vi "Three_Tote_Dashboard_Values.vi"(11 "3_Tote_Enable":bool=TRUE) -> ()   [LabVIEW 2014]
uses:
  General_VI/Global Var.vi
  <vilib>/Rock Robotics/Network Tables/SD Read Number.vi
panel:
  in  "Time _To_Drive_1_Tote":i32=8000
  in  "Extend_Flipper_Time":i32=500
  in  "Open_Infeed_time":i32=800
  # "Static Tunning Values"
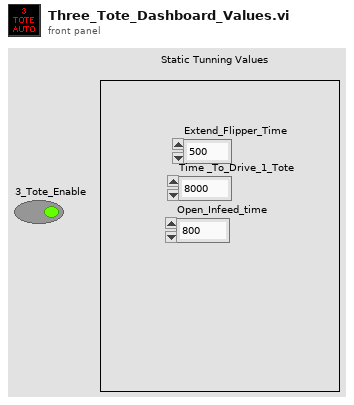
[diagram p1: front panel]
types:
  T1 = cluster{"Open_Infeed_time":i32, "Extend_Flipper_Time":i32, "Time _To_Drive_1_Tote":i32}
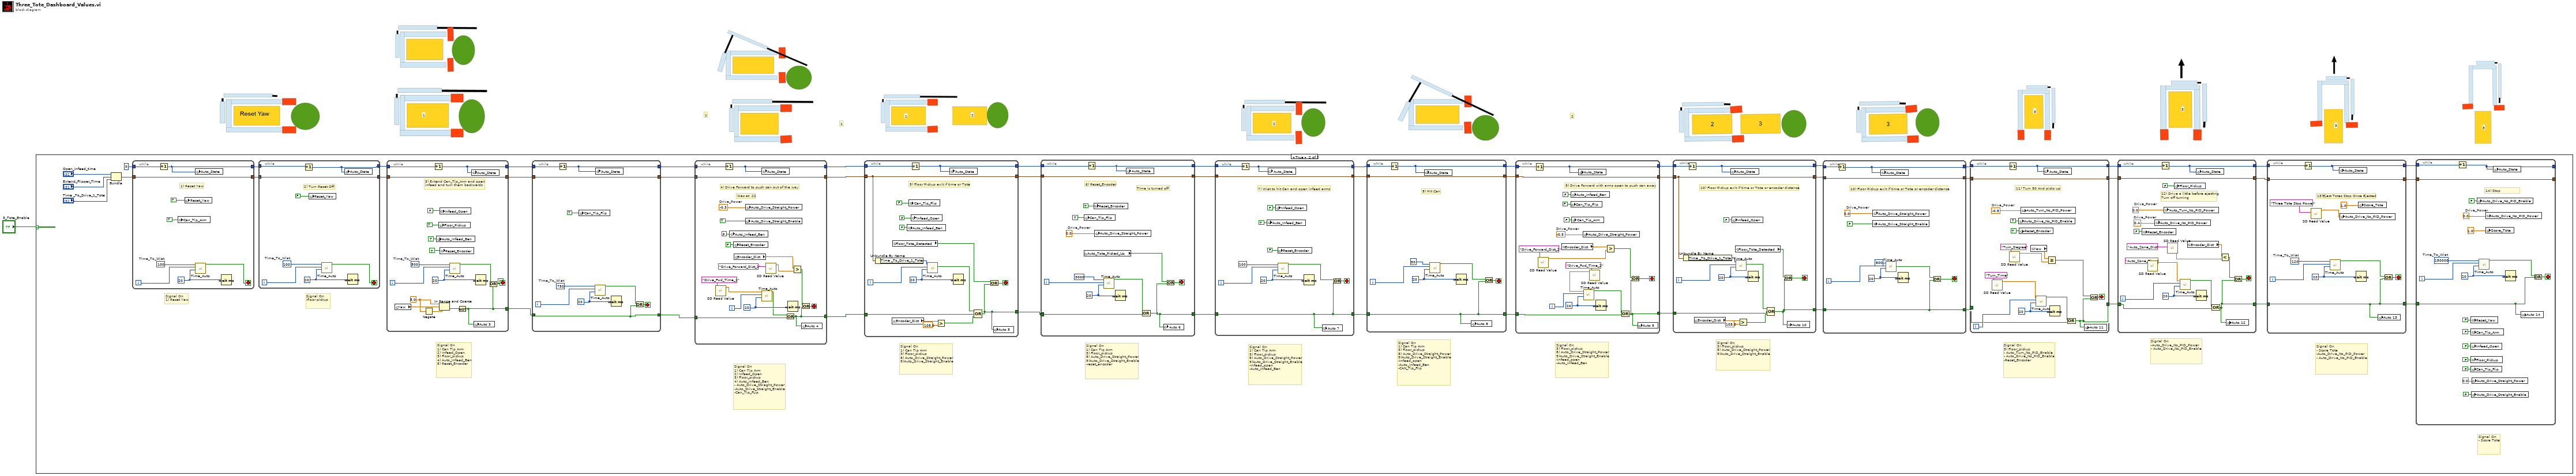
[diagram p0: block diagram]
diagram:
  # "3"
  # "3"
  # "3"
  # "3"
  # "2"
  # "2"
  # "2"
  # "1"
  # "1"
  # "1"
  # "1"
  n1 = case shown="True" "3_Tote_Enable" {
    frame False {
    }
    frame True {
      # "Signal On\n1) Can Tip Arm\n2) Infeed_Open\n3) Floor_pickup\n4) Auto_Infeed_Ben\n- Auto_Drive_Striaght_Power\n-Auto_Drive_Straight_Enable\n-Can_Tip_FLip"
      # "Signal On\n- Score Tote"
      # "Signal On\n- Score Tote\n-Auto_Drive_No_PID_Power\n- Auto_Drive_No_PID_Enable"
      # "Signal On\n-Auto_Drive_No_PID_Power\n- Auto_Drive_No_PID_Enable"
      # "Signal On\n3) Floor_pickup\n- Auto_Turn_No_PID_Enable\n- Auto_Drive_No_PID_Enable\n-Reset_Encoder"
      # "Signal On\n3) Floor_pickup\n8) Auto_Drive_Straight_Power\n9)Auto_Drive_Straight_Enable"
      # "Signal On\n3) Floor_pickup\n8) Auto_Drive_Straight_Power\n9)Auto_Drive_Straight_Enable\n-Infeed_open\n-Auto_Infeed_Ben"
      # "Signal On\n1) Can Tip Arm\n3) Floor_pickup\n8) Auto_Drive_Straight_Power\n9)Auto_Drive_Straight_Enable\n-Infeed_open\n-Auto_Infeed_Ben\n-CAN_Tip_Flip"
      # "Signal On\n1) Can Tip Arm\n3) Floor_pickup\n8) Auto_Drive_Straight_Power\n9)Auto_Drive_Straight_Enable\n-Infeed_open\n-Auto_Infeed_Ben"
      # "Signal On\n1) Can Tip Arm\n3) Floor_pickup\n8) Auto_Drive_Straight_Power\n9)Auto_Drive_Straight_Enable\n-reset_encoder"
      # "Signal On\n1) Can Tip Arm\n3) Floor_pickup\n8) Auto_Drive_Straight_Power\n9)Auto_Drive_Straight_Enable"
      # "Signal On\n1) Can Tip Arm\n2) Infeed_Open\n3) Floor_pickup\n4) Auto_Infeed_Ben\n5) Reset_Encoder"
      # "Signal On\n-floor pickup"
      # "Signal On\n1) Reset Yaw"
      n2 = Bundle("Open_Infeed_time"="Open_Infeed_time", "Extend_Flipper_Time"="Extend_Flipper_Time", "Time _To_Drive_1_Tote"="Time _To_Drive_1_Tote") -> (w39:T1)  [unwired: 1 in]
      n3 = while {
        tunnel: 0 -> [w271]
        tunnel: [w270] -> w48
        tunnel: w39 -> [w272]
        tunnel: [w272] -> w38
        i -> [w275]
        stop <- w277 stop-if-true
        w276 = u32 20 ("milliseconds to wait")
        w274 = 100  # Time_To_Wiat
        # "1) Reset Yaw"
        n4 = Increment(x=w271) -> (x+1=w270:i32)
        n5 = global write "Global Var.vi" "Can_Tip_Arm"(TRUE) -> ()
        n6 = global write "Global Var.vi" "Reset_Yaw"(TRUE) -> ()
        n7 = global write "Global Var.vi" "Auto_State"(w270) -> ()
        n8 = call "Time_Auto.vi"("Sample_Time"=w276, "Counter"=w275, "Time_to_wait"=w274) -> ("Boolean"=w277:bool)  [unwired: 8 in]
        n9 = Wait (ms)(milliseconds to wait=w276) -> ()  [unwired: 1 out]
      }
      n10 = while {
        tunnel: w48 -> [w262]
        tunnel: [w261] -> w47
        tunnel: w38 -> [w263]
        tunnel: [w263] -> w37
        i -> [w266]
        stop <- w268 stop-if-true
        w267 = u32 20 ("milliseconds to wait")
        w265 = 100  # Time_To_Wiat
        # "2) Turn Reset Off"
        n11 = Increment(x=w262) -> (x+1=w261:i32)
        n12 = global write "Global Var.vi" "Reset_Yaw"(FALSE) -> ()
        n13 = call "Time_Auto.vi"("Sample_Time"=w267, "Counter"=w266, "Time_to_wait"=w265) -> ("Boolean"=w268:bool)  [unwired: 8 in]
        n14 = global write "Global Var.vi" "Auto_State"(w261) -> ()
        n15 = Wait (ms)(milliseconds to wait=w267) -> ()  [unwired: 1 out]
      }
      n16 = while {
        tunnel: w47 -> [w256]
        tunnel: [w255] -> w11
        tunnel: w37 -> [w257]
        tunnel: [w257] -> w12
        tunnel: [w245] -> w14
        i -> [w259]
        stop <- w247 stop-if-true
        w251 = 5.0 ("upper limit")
        w260 = u32 20 ("milliseconds to wait")
        w258 = 500  # Time_To_Wiat
        # "3) Extend Can_Tip_Arm and open \ninfeed and turn them backwards"
        n17 = global read "Global Var.vi" "Yaw"() -> (w253:dbl)
        n18 = Negate(x=w251) -> (-x=w252:dbl)
        n19 = Increment(x=w256) -> (x+1=w255:i32)
        n20 = global write "Global Var.vi" "Auto_Infeed_Ben"(TRUE) -> ()
        n21 = global write "Global Var.vi" "Floor_Pickup"(TRUE) -> ()
        n22 = In Range and Coerce(upper limit=w251, x=w253, lower limit=w252) -> (In Range?=w250:bool)  [unwired: 1 out]
        n23 = global write "Global Var.vi" "Infeed_Open"(FALSE) -> ()
        n24 = global write "Global Var.vi" "Reset_Encoder"(TRUE) -> ()
        n25 = call "Time_Auto.vi"("Sample_Time"=w260, "Counter"=w259, "Time_to_wait"=w258) -> ("Boolean"=w246:bool)  [unwired: 8 in]
        n26 = Not(x=w250) -> (.not. x?=w245:bool)
        n27 = global write "Global Var.vi" "Auto_State"(w255) -> ()
        n28 = global write "Global Var.vi" "Auto 3"(w245) -> ()
        n29 = Wait (ms)(milliseconds to wait=w260) -> ()  [unwired: 1 out]
        n30 = Or(x=w246, y=w245) -> (x .or. y?=w247:bool)
      }
      n31 = while {
        tunnel: w11 -> [w66]
        tunnel: [w65] -> w10
        tunnel: w12 -> [w67]
        tunnel: [w67] -> w9
        tunnel: w14 -> [w61]
        tunnel: [w61] -> w13
        i -> [w69]
        stop <- w64 stop-if-true
        w70 = u32 20 ("milliseconds to wait")
        w68 = 750  # Time_To_Wiat
        n32 = Increment(x=w66) -> (x+1=w65:i32)
        n33 = global write "Global Var.vi" "Can_Tip_Flip"(TRUE) -> ()
        n34 = call "Time_Auto.vi"("Sample_Time"=w70, "Counter"=w69, "Time_to_wait"=w68) -> ("Boolean"=w62:bool)  [unwired: 8 in]
        n35 = global write "Global Var.vi" "Auto_State"(w65) -> ()
        n36 = Wait (ms)(milliseconds to wait=w70) -> ()  [unwired: 1 out]
        n37 = Or(x=w62, y=w61) -> (x .or. y?=w64:bool)
      }
      n38 = while {
        tunnel: w10 -> [w240]
        tunnel: [w239] -> w33
        tunnel: w9 -> [w241]
        tunnel: [w241] -> w32
        tunnel: w13 -> [w233]
        tunnel: [w230] -> w31
        i -> [w242]
        stop <- w232 stop-if-true
        w238 = -0.3  # Drive_Power
        w243 = u32 20 ("milliseconds to wait")
        # "Was at .22"
        # "4) Drive Forward to push can out of the way"
        n39 = call-poly <vilib>:"SD Read Value.vi"("Name"="Drive_Fwd_Time_1") -> ("Numeric"=w225:dbl)  [unwired: 8 in, 2 out]
        n40 = Increment(x=w240) -> (x+1=w239:i32)
        n41 = global write "Global Var.vi" "Auto_Infeed_Ben"(FALSE) -> ()
        n42 = global write "Global Var.vi" "Reset_Encoder"(FALSE ("Reset_Encoder")) -> ()
        n43 = global read "Global Var.vi" "Encoder_Dist"() -> (w235:dbl)
        n44 = global write "Global Var.vi" "Auto_Drive_Straight_Enable"(TRUE) -> ()
        n45 = global write "Global Var.vi" "Auto_Drive_Straight_Power"(w238) -> ()
        n46 = call "Time_Auto.vi"("Sample_Time"=w243, "Counter"=w242, "Time_to_wait"=w225) -> ("Boolean"=w234:bool)  [unwired: 8 in]
        n47 = global write "Global Var.vi" "Auto_State"(w239) -> ()
        n48 = call-poly <vilib>:"SD Read Value.vi"("Name"="Drive_Forward_Dist_1") -> ("Numeric"=w227:dbl)  [unwired: 8 in, 2 out]
        n49 = Or(x=w234, y=w233) -> (x .or. y?=w230:bool)
        n50 = Wait (ms)(milliseconds to wait=w243) -> ()  [unwired: 1 out]
        n51 = Greater?(x=w235, y=w227) -> (0:w231:bool)
        n52 = Or(x=w231, y=w230) -> (x .or. y?=w232:bool)
        n53 = global write "Global Var.vi" "Auto 4"(w230) -> ()
      }
      n54 = while {
        tunnel: w33 -> [w222]
        tunnel: [w221] -> w30
        tunnel: w32 -> [w220]
        tunnel: [w220] -> w29
        tunnel: w31 -> [w218]
        tunnel: [w208] -> w2
        i -> [w223]
        stop <- w214 stop-if-true
        w224 = u32 20 ("milliseconds to wait")
        # "5) Floor Pickup exit if time or Tote"
        n55 = Unbundle By Name(w220) -> ("Time _To_Drive_1_Tote"=w219:i32)
        n56 = global read "Global Var.vi" "Encoder_Dist"() -> (w212:dbl)
        n57 = global read "Global Var.vi" "Floor_Tote_Detected"() -> (w213:bool)
        n58 = global write "Global Var.vi" "Auto_Infeed_Ben"(FALSE) -> ()
        n59 = global write "Global Var.vi" "Can_Tip_Flip"(FALSE) -> ()
        n60 = Increment(x=w222) -> (x+1=w221:i32)
        n61 = global write "Global Var.vi" "Infeed_Open"(FALSE) -> ()
        n62 = call "Time_Auto.vi"("Sample_Time"=w224, "Counter"=w223, "Time_to_wait"=w219) -> ("Boolean"=w217:bool)  [unwired: 8 in]
        n63 = Greater?(x=w212, y=105.0) -> (0:w211:bool)
        n64 = global write "Global Var.vi" "Auto_State"(w221) -> ()
        n65 = Wait (ms)(milliseconds to wait=w224) -> ()  [unwired: 1 out]
        n66 = Compound Arithmetic op=OR(w217, w218, w211) -> (w208:bool)
        n67 = Or(x=w213, y=w208) -> (x .or. y?=w214:bool)
        n68 = global write "Global Var.vi" "Auto 5"(w208) -> ()
      }
      n69 = while {
        tunnel: w30 -> [w101]
        tunnel: [w100] -> w15
        tunnel: w29 -> [w99]
        tunnel: [w99] -> w22
        tunnel: w2 -> [_]
        tunnel: [w91] -> w28
        tunnel: w2 -> [w92]
        i -> [w102]
        stop <- w98 stop-if-true
        w94 = 0.0  # Drive_Power
        w103 = u32 20 ("milliseconds to wait")
        # "TIme is turned off"
        # "6) Reset_Encoder"
        n70 = global read "Global Var.vi" "Auto_Tote_Picked_Up"() -> (w95:bool)
        n71 = global write "Global Var.vi" "Can_Tip_Flip"(TRUE) -> ()
        n72 = Increment(x=w101) -> (x+1=w100:i32)
        n73 = global write "Global Var.vi" "Reset_Encoder"(TRUE) -> ()
        n74 = global write "Global Var.vi" "Auto_Drive_Straight_Power"(w94) -> ()
        n75 = call "Time_Auto.vi"("Sample_Time"=w103, "Counter"=w102, "Time_to_wait"=3000) -> ("Boolean"=w93:bool)  [unwired: 8 in]
        n76 = Wait (ms)(milliseconds to wait=w103) -> ()  [unwired: 1 out]
        n77 = global write "Global Var.vi" "Auto_State"(w100) -> ()
        n78 = Compound Arithmetic op=OR(w93, w92) -> (w91:bool)
        n79 = global write "Global Var.vi" "Auto 6"(w91) -> ()
        n80 = Or(x=w95, y=w91) -> (x .or. y?=w98:bool)
      }
      n81 = while {
        tunnel: [w205] -> w46
        tunnel: w28 -> [w196]
        tunnel: [w196] -> w27
        tunnel: w22 -> [w198]
        tunnel: [w198] -> w21
        tunnel: w15 -> [w197]
        i -> [w206]
        stop <- w203 stop-if-true
        w207 = u32 20 ("milliseconds to wait")
        # "7) Wiat to hit Can and open infeed arms"
        n82 = Increment(x=w197) -> (x+1=w205:i32)
        n83 = global write "Global Var.vi" "Auto_Infeed_Ben"(TRUE) -> ()
        n84 = global write "Global Var.vi" "Auto_State"(w205) -> ()
        n85 = global write "Global Var.vi" "Infeed_Open"(FALSE ("Infeed_Open")) -> ()
        n86 = global write "Global Var.vi" "Reset_Encoder"(FALSE) -> ()
        n87 = call "Time_Auto.vi"("Sample_Time"=w207, "Counter"=w206, "Time_to_wait"=100) -> ("Boolean"=w202:bool)  [unwired: 8 in]
        n88 = Wait (ms)(milliseconds to wait=w207) -> ()  [unwired: 1 out]
        n89 = global write "Global Var.vi" "Auto 7"(w196) -> ()
        n90 = Or(x=w202, y=w196) -> (x .or. y?=w203:bool)
      }
      n91 = while {
        tunnel: w46 -> [w193]
        tunnel: [w192] -> w26
        tunnel: w27 -> [w187]
        tunnel: [w187] -> w24
        tunnel: w21 -> [w189]
        tunnel: [w189] -> w20
        i -> [w194]
        stop <- w191 stop-if-true
        w195 = u32 20 ("milliseconds to wait")
        # "8) HIt Can"
        n92 = Increment(x=w193) -> (x+1=w192:i32)
        n93 = global write "Global Var.vi" "Auto_State"(w192) -> ()
        n94 = call "Time_Auto.vi"("Sample_Time"=w195, "Counter"=w194, "Time_to_wait"=50) -> ("Boolean"=w190:bool)  [unwired: 8 in]
        n95 = Wait (ms)(milliseconds to wait=w195) -> ()  [unwired: 1 out]
        n96 = global write "Global Var.vi" "Auto 8"(w187) -> ()
        n97 = Or(x=w190, y=w187) -> (x .or. y?=w191:bool)
      }
      n98 = while {
        tunnel: [w86] -> w25
        tunnel: w26 -> [w85]
        tunnel: w24 -> [w83]
        tunnel: [w77] -> w23
        tunnel: w20 -> [w79]
        tunnel: [w79] -> w19
        i -> [w88]
        stop <- w87 stop-if-true
        w76 = -0.3  # Drive_Power
        w89 = u32 20 ("milliseconds to wait")
        # "9) Drive Forward with arms open to push can away"
        n99 = Increment(x=w85) -> (x+1=w86:i32)
        n100 = call-poly <vilib>:"SD Read Value.vi"("Name"="Drive_Forward_Dist_2") -> ("Numeric"=w74:dbl)  [unwired: 8 in, 2 out]
        n101 = global read "Global Var.vi" "Encoder_Dist"() -> (w82:dbl)
        n102 = global write "Global Var.vi" "Can_Tip_Flip"(FALSE ("Infeed_Open")) -> ()
        n103 = global write "Global Var.vi" "Auto_Infeed_Ben"(FALSE) -> ()
        n104 = global write "Global Var.vi" "Can_Tip_Arm"(FALSE ("Infeed_Open")) -> ()
        n105 = global write "Global Var.vi" "Auto_State"(w86) -> ()
        n106 = global write "Global Var.vi" "Auto_Drive_Straight_Power"(w76) -> ()
        n107 = call-poly <vilib>:"SD Read Value.vi"("Name"="Drive_Fwd_Time_2") -> ("Numeric"=w72:dbl)  [unwired: 8 in, 2 out]
        n108 = call "Time_Auto.vi"("Sample_Time"=w89, "Counter"=w88, "Time_to_wait"=w72) -> ("Boolean"=w84:bool)  [unwired: 8 in]
        n109 = Wait (ms)(milliseconds to wait=w89) -> ()  [unwired: 1 out]
        n110 = Greater?(x=w82, y=w74) -> (0:w81:bool)
        n111 = Compound Arithmetic op=OR(w84, w83) -> (w77:bool)
        n112 = Or(x=w81, y=w77) -> (x .or. y?=w87:bool)
        n113 = global write "Global Var.vi" "Auto 9"(w77) -> ()
      }
      n114 = while {
        tunnel: [w182] -> w8
        tunnel: [w172] -> w5
        tunnel: w25 -> [w179]
        tunnel: w23 -> [w176]
        tunnel: w19 -> [w174]
        tunnel: [w174] -> w3
        i -> [w185]
        stop <- w184 stop-if-true
        w186 = u32 20 ("milliseconds to wait")
        # "10) Floor Pickup exit if time or Tote or encoder distance"
        n115 = Unbundle By Name(w174) -> ("Time _To_Drive_1_Tote"=w181:i32)
        n116 = Increment(x=w179) -> (x+1=w182:i32)
        n117 = global read "Global Var.vi" "Encoder_Dist"() -> (w177:dbl)
        n118 = global write "Global Var.vi" "Auto_State"(w182) -> ()
        n119 = global write "Global Var.vi" "Infeed_Open"(FALSE ("Infeed_Open")) -> ()
        n120 = global read "Global Var.vi" "Floor_Tote_Detected"() -> (w183:bool)
        n121 = call "Time_Auto.vi"("Sample_Time"=w186, "Counter"=w185, "Time_to_wait"=w181) -> ("Boolean"=w180:bool)  [unwired: 8 in]
        n122 = Greater?(x=w177, y=105.0) -> (0:w175:bool)
        n123 = Wait (ms)(milliseconds to wait=w186) -> ()  [unwired: 1 out]
        n124 = Compound Arithmetic op=OR(w180, w176, w175) -> (w172:bool)
        n125 = Or(x=w183, y=w172) -> (x .or. y?=w184:bool)
        n126 = global write "Global Var.vi" "Auto 10"(w172) -> ()
      }
      n127 = while {
        tunnel: [w58] -> w7
        tunnel: w8 -> [w57]
        tunnel: w3 -> [w56]
        tunnel: [w56] -> w6
        tunnel: w5 -> [w53]
        tunnel: [w53] -> w4
        i -> [w59]
        stop <- w55 stop-if-true
        w51 = 0.0  # Drive_Power
        w60 = u32 20 ("milliseconds to wait")
        # "10) Floor Pickup exit if time or Tote or encoder distance"
        n128 = Increment(x=w57) -> (x+1=w58:i32)
        n129 = global write "Global Var.vi" "Auto_Drive_Straight_Enable"(FALSE) -> ()
        n130 = global write "Global Var.vi" "Auto_Drive_Straight_Power"(w51) -> ()
        n131 = global write "Global Var.vi" "Auto_State"(w58) -> ()
        n132 = call "Time_Auto.vi"("Sample_Time"=w60, "Counter"=w59, "Time_to_wait"=800) -> ("Boolean"=w54:bool)  [unwired: 8 in]
        n133 = Wait (ms)(milliseconds to wait=w60) -> ()  [unwired: 1 out]
        n134 = Or(x=w54, y=w53) -> (x .or. y?=w55:bool)
      }
      n135 = while {
        tunnel: w7 -> [w170]
        tunnel: [w169] -> w45
        tunnel: w4 -> [w162]
        tunnel: [w158] -> w36
        tunnel: w6 -> [w166]
        tunnel: [w166] -> w18
        i -> [w163]
        stop <- w160 stop-if-true
        w164 = u32 20 ("milliseconds to wait")
        w168 = -0.5  # Drive_Power
        # "11) Turn 90 And picks up"
        n136 = call-poly <vilib>:"SD Read Value.vi"("Name"="Turn_Time") -> ("Numeric"=w154:dbl)  [unwired: 8 in, 2 out]
        n137 = Increment(x=w170) -> (x+1=w169:i32)
        n138 = call-poly <vilib>:"SD Read Value.vi"("Name"="Turn_Degree") -> ("Numeric"=w155:dbl)  [unwired: 8 in, 2 out]
        n139 = global write "Global Var.vi" "Auto_Drive_No_PID_Enable"(TRUE ("Auto_Drive_No_PID_Enable")) -> ()
        n140 = global write "Global Var.vi" "Reset_Encoder"(TRUE ("Reset_Encoder")) -> ()
        n141 = global write "Global Var.vi" "Auto_Turn_No_PID_Power"(w168) -> ()
        n142 = global read "Global Var.vi" "Yaw"() -> (w171:dbl)
        n143 = call "Time_Auto.vi"("Sample_Time"=w164, "Counter"=w163, "Time_to_wait"=w154) -> ("Boolean"=w161:bool)  [unwired: 8 in]
        n144 = global write "Global Var.vi" "Auto_State"(w169) -> ()
        n145 = Greater Or Equal?(x=w171, y=w155) -> (x >= y?=w159:bool)
        n146 = Wait (ms)(milliseconds to wait=w164) -> ()  [unwired: 1 out]
        n147 = Compound Arithmetic op=OR(w161, w162) -> (w158:bool)
        n148 = global write "Global Var.vi" "Auto 11"(w158) -> ()
        n149 = Or(x=w159, y=w158) -> (x .or. y?=w160:bool)
      }
      n150 = while {
        tunnel: w45 -> [w150]
        tunnel: [w149] -> w44
        tunnel: w36 -> [w144]
        tunnel: [w139] -> w35
        tunnel: w18 -> [w147]
        tunnel: [w147] -> w17
        i -> [w152]
        stop <- w141 stop-if-true
        w148 = 0.0  # Drive_Power
        w151 = 0.4  # Drive_Power
        w153 = u32 20 ("milliseconds to wait")
        # "12) Drive a little before ejecting\nTurn off turning"
        n151 = global write "Global Var.vi" "Reset_Encoder"(FALSE ("Reset_Encoder")) -> ()
        n152 = call-poly <vilib>:"SD Read Value.vi"("Name"="Auto_Zone_Time") -> ("Numeric"=w136:dbl)  [unwired: 8 in, 2 out]
        n153 = global write "Global Var.vi" "Auto_Drive_No_PID_Power"(w151) -> ()
        n154 = Increment(x=w150) -> (x+1=w149:i32)
        n155 = global write "Global Var.vi" "Auto_Turn_No_PID_Power"(w148) -> ()
        n156 = call-poly <vilib>:"SD Read Value.vi"("Name"="Auto_Zone_Dist") -> ("Numeric"=w135:dbl)  [unwired: 8 in, 2 out]
        n157 = global write "Global Var.vi" "Floor_Pickup"(FALSE) -> ()
        n158 = call "Time_Auto.vi"("Sample_Time"=w153, "Counter"=w152, "Time_to_wait"=w136) -> ("Boolean"=w145:bool)  [unwired: 8 in]
        n159 = global read "Global Var.vi" "Encoder_Dist"() -> (w142:dbl)
        n160 = global write "Global Var.vi" "Auto_State"(w149) -> ()
        n161 = Wait (ms)(milliseconds to wait=w153) -> ()  [unwired: 1 out]
        n162 = Compound Arithmetic op=OR(w145, w144) -> (w139:bool)
        n163 = Less?(x=w142, y=w135) -> (x < y?=w140:bool)
        n164 = global write "Global Var.vi" "Auto 12"(w139) -> ()
        n165 = Or(x=w140, y=w139) -> (x .or. y?=w141:bool)
      }
      n166 = while {
        tunnel: w44 -> [w130]
        tunnel: [w129] -> w43
        tunnel: w35 -> [w125]
        tunnel: [w125] -> w34
        tunnel: w17 -> [w128]
        tunnel: [w128] -> w16
        i -> [w133]
        stop <- w127 stop-if-true
        w134 = u32 20 ("milliseconds to wait")
        w132 = 120  # Time_To_Wiat
        # "13)Eject Totes Stop Once Ejected"
        n167 = Increment(x=w130) -> (x+1=w129:i32)
        n168 = call-poly <vilib>:"SD Read Value.vi"("Name"="Three Tote Stop Power") -> ("Numeric"=w123:dbl)  [unwired: 8 in, 2 out]
        n169 = call "Time_Auto.vi"("Sample_Time"=w134, "Counter"=w133, "Time_to_wait"=w132) -> ("Boolean"=w126:bool)  [unwired: 8 in]
        n170 = global write "Global Var.vi" "Auto_State"(w129) -> ()
        n171 = global write "Global Var.vi" "Auto_Drive_No_PID_Power"(w123) -> ()
        n172 = Wait (ms)(milliseconds to wait=w134) -> ()  [unwired: 1 out]
        n173 = global write "Global Var.vi" "Score_Tote"(1.0) -> ()
        n174 = global write "Global Var.vi" "Auto 13"(w125) -> ()
        n175 = Or(x=w126, y=w125) -> (x .or. y?=w127:bool)
      }
      n176 = while {
        tunnel: w43 -> [w118]
        tunnel: [w117] -> _
        tunnel: w34 -> [w104]
        tunnel: w16 -> [w107]
        tunnel: [w107] -> _
        i -> [w121]
        stop <- w106 stop-if-true
        w115 = 0.0  # Drive_Power
        w122 = u32 20 ("milliseconds to wait")
        w120 = 150000  # Time_To_Wiat
        # "14) Stop"
        n177 = Increment(x=w118) -> (x+1=w117:i32)
        n178 = global write "Global Var.vi" "Reset_Yaw"(FALSE ("Reset_Yaw")) -> ()
        n179 = global write "Global Var.vi" "Can_Tip_Arm"(FALSE ("Can_Tip_Arm")) -> ()
        n180 = global write "Global Var.vi" "Infeed_Open"(FALSE ("Infeed_Open")) -> ()
        n181 = global write "Global Var.vi" "Floor_Pickup"(FALSE ("Floor_Pickup")) -> ()
        n182 = global write "Global Var.vi" "Can_Tip_Flip"(FALSE ("Can_Tip_Flip")) -> ()
        n183 = global write "Global Var.vi" "Auto_Drive_Straight_Enable"(FALSE ("Auto_Drive_Straight_Enable")) -> ()
        n184 = global write "Global Var.vi" "Auto_Drive_Straight_Power"(0.0 ("Auto_Drive_Straight_Power")) -> ()
        n185 = global write "Global Var.vi" "Auto_Drive_No_PID_Enable"(FALSE ("Auto_Drive_No_PID_Enable")) -> ()
        n186 = call "Time_Auto.vi"("Sample_Time"=w122, "Counter"=w121, "Time_to_wait"=w120) -> ("Boolean"=w105:bool)  [unwired: 8 in]
        n187 = global write "Global Var.vi" "Score_Tote"(1.0) -> ()
        n188 = global write "Global Var.vi" "Auto_Drive_No_PID_Power"(w115) -> ()
        n189 = global write "Global Var.vi" "Auto_State"(w117) -> ()
        n190 = Wait (ms)(milliseconds to wait=w122) -> ()  [unwired: 1 out]
        n191 = global write "Global Var.vi" "Auto 14"(w104) -> ()
        n192 = Or(x=w105, y=w104) -> (x .or. y?=w106:bool)
      }
    }
  }
